vi "Register.vi"(8 "error in (no error)":errorcluster, 11 "object in":refnum<class "EventMsg.lvclass">) -> (0 "error out":errorcluster, 2 "Event Registration Refnum":refnum<event-registration>, 3 "object out":refnum<class "EventMsg.lvclass">)   [LabVIEW 2014, in "EventMsg.lvclass"]
uses:
  EventMsg.lvclass
  EventMsg.lvclass/EventMsg.ctl
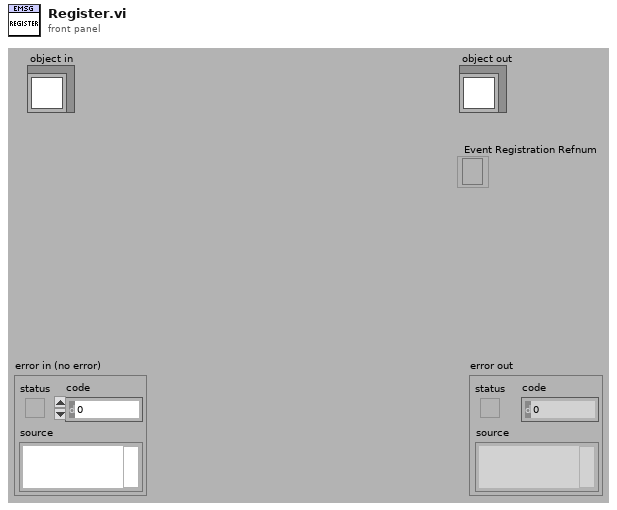
[diagram p1: front panel]
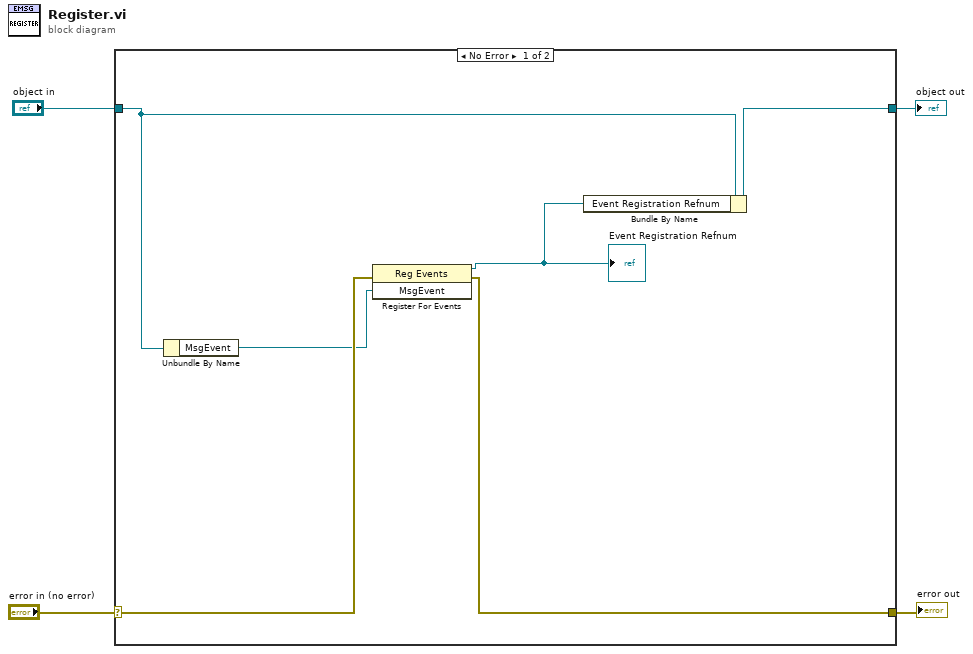
[diagram p0: block diagram]
diagram:
  n1 = case shown="No Error" "error in (no error)" {
    selector: "error in (no error)" -> [w10 w12]
    tunnel: [w9 w12] -> w3
    tunnel: [w8 w11] -> w1
    tunnel: "object in" -> [w7 w11]
    frame No Error {
      n2 = Unbundle By Name(w7) -> ("MsgEvent"=w5:refnum<user-event>)
      n3 = register-events(error in=w10, w5) -> (reference out=w6:refnum<event-registration>, error out=w9:errorcluster)  [unwired: 1 in]
      "Event Registration Refnum" <- w6
      n4 = Bundle By Name(cluster=w7, "Event Registration Refnum"=w6) -> (w8:refnum<class "EventMsg.lvclass">)
    }
    frame Error {
    }
  }
  "error out" <- w3
  "object out" <- w1
